vi "启动测试.vi"   [LabVIEW 2016, in "EXO2-Sonde.lvlib"]
uses:
  EXO2-Sonde.lvlib
  Var/Input Var.vi
types:
  T1 = enum16{"init", "run", "test", "storage", "stop", "end"}
  T2 = cluster{"Temp":dbl, "SpCond":dbl, "Cond":dbl, "Sal":dbl, "TDS":dbl, "pH":dbl, "pH mV":dbl, "orp":dbl, "ODO %":dbl, "ODO mg/L":dbl, "Turb":dbl, "Chl":dbl, "Algae":dbl, "Depth":dbl}
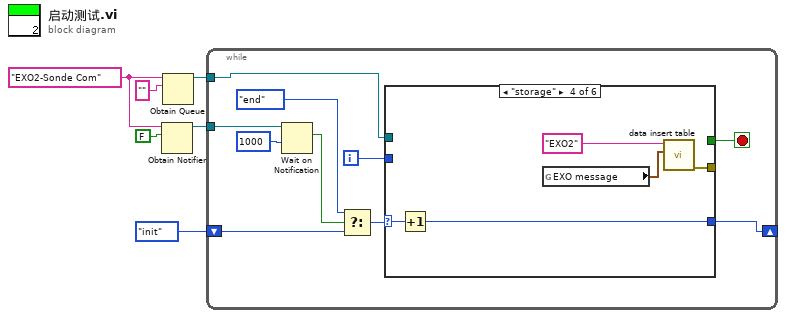
[diagram p0: block diagram]
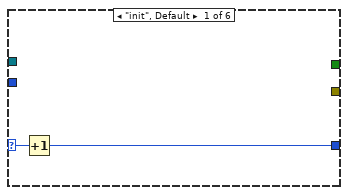
[diagram p2: hidden frame]
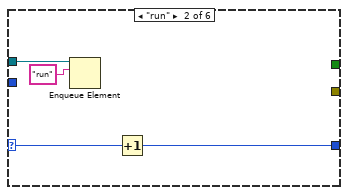
[diagram p3: hidden frame]
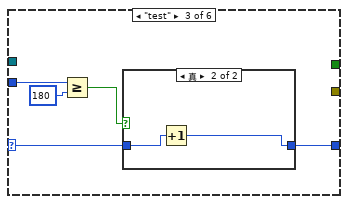
[diagram p4: hidden frame]
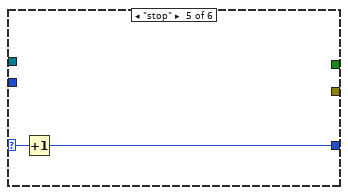
[diagram p6: hidden frame]
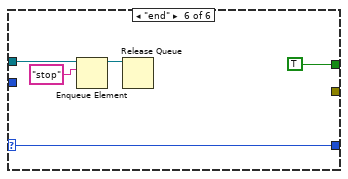
[diagram p7: hidden frame]
diagram:
  w3 = "EXO2-Sonde Com" ("名称（未命名）")
  n1 = Obtain Notifier(name (unnamed)=w3, notification data type=FALSE) -> (notifier out=w1:refnum<notifier>)  [unwired: 2 in, 2 out]
  n2 = Obtain Queue(name (unnamed)=w3, element data type="") -> (queue out=w4:refnum<queue>)  [unwired: 3 in, 2 out]
  n3 = while {
    shift-right: [w15] -> _
    shift-left: T1."init" ("枚举") -> [w8]
    tunnel: w4 -> [w16]
    tunnel: w1 -> [w12]
    i -> [w14]
    stop <- w13 stop-if-true
    n4 = Wait on Notification(notifier=w12, timeout in ms (-1)=1000 ("超时毫秒(-1)")) -> (notification=w9:bool)  [unwired: 2 in, 3 out]
    n5 = Select(t=T1."end", s=w9, f=w8) -> (s? t:f=w10:T1)
    n6 = case shown="\"storage\"" w10 {
      selector: w10 -> [w18 w20 w27 w35 w37 w42]
      tunnel: w16 -> [_ w21 _ _ _ w39]
      tunnel: [w17 w19 w26 w34 w36 w42] -> w15
      tunnel: w14 -> [_ _ w25 _ _ _]
      tunnel: [_ _ _ w31 _ _] -> _
      tunnel: [_ _ _ _ _ TRUE] -> w13
      frame "init", Default {
        n7 = Increment(x=w18) -> (x+1=w17:T1)
      }
      frame "run" {
        n8 = Enqueue Element(queue=w21, element="run" ("元素")) -> ()  [unwired: 2 in, 3 out]
        n9 = Increment(x=w20) -> (x+1=w19:T1)
      }
      frame "test" {
        n10 = Greater Or Equal?(x=w25, y=180) -> (x >= y?=w23:bool)
        n11 = case shown="真" w23 {
          tunnel: w27 -> [w28 w30]
          tunnel: [w28 w29] -> w26
          frame False {
          }
          frame True {
            n12 = Increment(x=w30) -> (x+1=w29:T1)
          }
        }
      }
      frame "storage" {
        n13 = Increment(x=w35) -> (x+1=w34:T1)
        n14 = global read "Input Var.vi" "EXO message"() -> (w33:T2)
        n15 = call "data insert table.vi"("EXO message"=w33, "table"="EXO2") -> ("error out"=w31:errorcluster)  [unwired: 9 in]
      }
      frame "stop" {
        n16 = Increment(x=w37) -> (x+1=w36:T1)
      }
      frame "end" {
        n17 = Enqueue Element(queue=w39, element="stop" ("元素")) -> (queue out=w38:refnum<queue>)  [unwired: 2 in, 2 out]
        n18 = Release Queue(queue=w38) -> ()  [unwired: 2 in, 3 out]
      }
    }
  }
